vi "test_Double (Missing).vi"(8 "error in (no error)":errorcluster, 11 "TestCase in":refnum<class "Read File Tests.lvclass">) -> (0 "error out":errorcluster, 3 "TestCase out":refnum<class "Read File Tests.lvclass">)   [LabVIEW 2017, in "Read File Tests.lvclass"]
uses:
  Read File Tests.lvclass
  Read File Tests.lvclass/Read File Tests.ctl
  Read/Read Section - Double.vi
  <vilib>/addons/_JKI Toolkits/VI Tester/TestCase.llb/TestCase.lvclass
  TSC File IO.lvlib
  C:/Program Files (x86)/National Instruments/LabVIEW 2017/vi.lib/addons/_JKI Toolkits/VI Tester/TestCase.llb/TestCase.lvclass
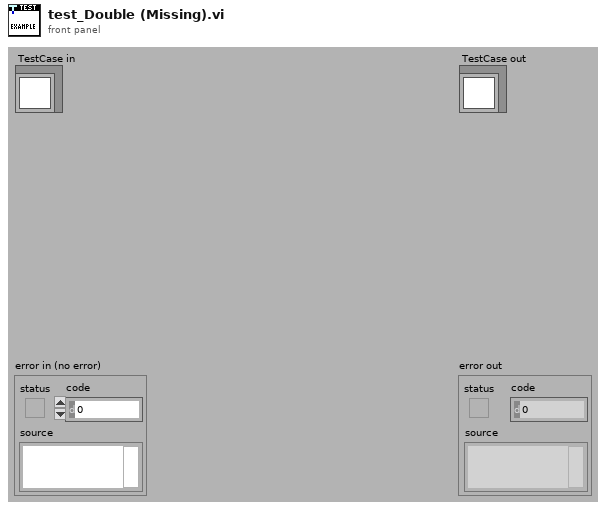
[diagram p1: front panel]
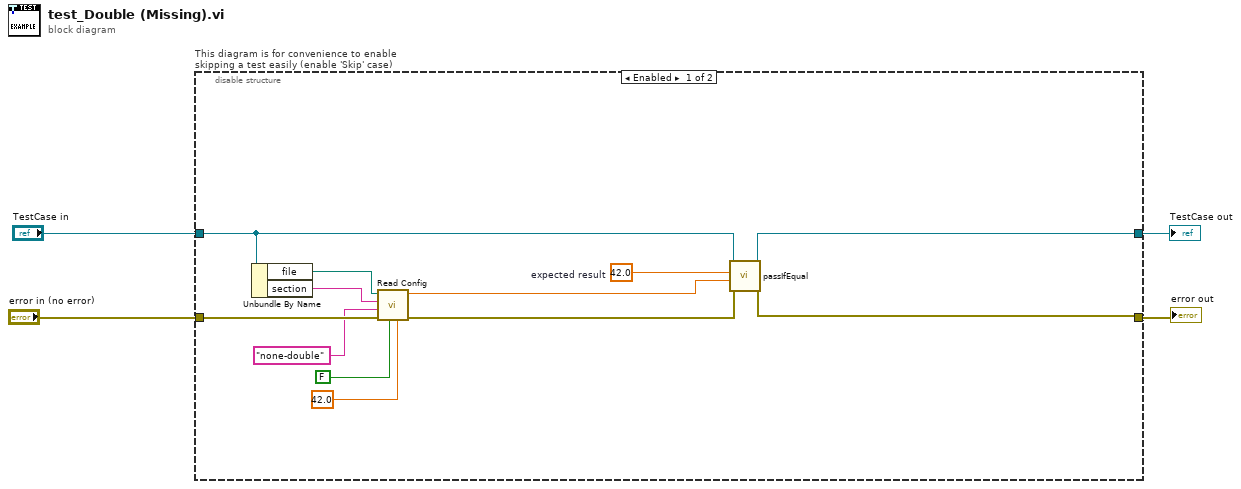
[diagram p0: block diagram]
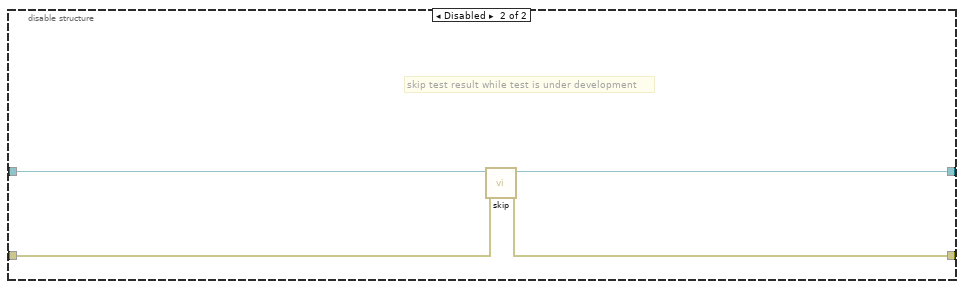
[diagram p2: hidden frame]
diagram:
  n1 = disable-structure "This diagram is for convenience to enable skipping a test easily (enable 'Skip' case)" shown="Enabled" {
    disable-tunnel: "TestCase in" -> [w13 w20]
    disable-tunnel: [w15 w18] -> w1
    disable-tunnel: [w14 w19] -> w3
    disable-tunnel: "error in (no error)" -> [w12 w17]
    frame Enabled {
      w16 = 42.0  # expected result
      n2 = Unbundle By Name(w13) -> ("file"=w10:path, "section"=w9:string)
      n3 = call-poly "Read Config.vi"("Default"=42.0, "Create file if not found? (T)"=FALSE, "error in (no error)"=w12, "key"="none-double", "section"=w9, "Path"=w10) -> ("error out"=w11:errorcluster, "value"=w8:dbl)  [unwired: 4 in]
      n4 = call-dynamic "passIfEqual.vi"("error in (no error)"=w11, "y"=w8, "x"=w16, "TestCase in"=w13) -> ("error out"=w14:errorcluster, "TestCase out"=w15:refnum<class "Read File Tests.lvclass">)  [unwired: 6 in]
    }
    frame Disabled {
      # "skip test result while test is under development"
      n5 = call <vilib>:"skip.vi"("error in (no error)"=w17, "TestCase in"=w20) -> ("error out"=w19:errorcluster, "TestCase out"=w18:refnum<class "Read File Tests.lvclass">)  [unwired: 8 in]
    }
  }
  "error out" <- w3
  "TestCase out" <- w1
